vi "Process.vi"(0 "reference in":refnum<class "Reporter.lvclass">, 5 "error in (no error)":errorcluster) -> (14 "reference out":refnum<class "Reporter.lvclass">, 19 "error out":errorcluster)   [LabVIEW 2018, in "Reporter.lvclass"]
uses:
  Reporter.lvclass
  controls/IO Signal List.ctl
  BKP-891 LCR Meter_class/BKP-891 LCR Meter.lvclass
  BKP-911x Power Supply_class/BKP-911x Power Supply.lvclass
  NI-DAQmx_class/NI-DAQmx.lvclass
panel:
  in  "Signal MCLB":i32(listbox)
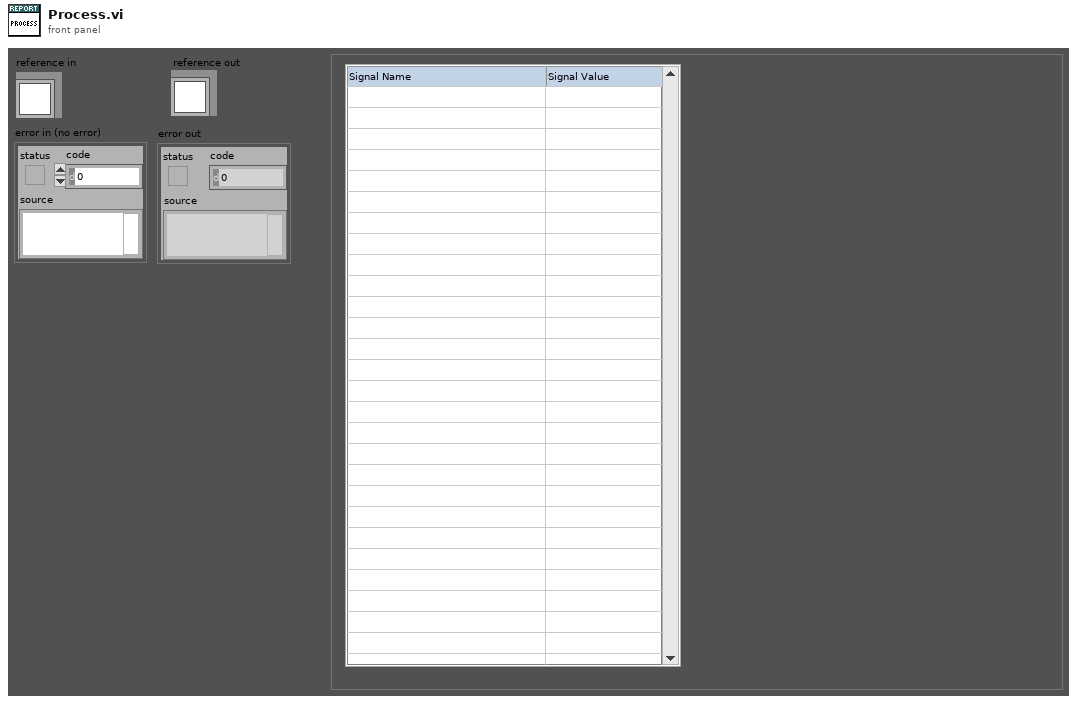
[diagram p1: front panel]
types:
  T1 = typedef "IO Signal List.ctl" = enum16{"Timestamp", "PSU_FB_U_VDC", "PSU_FB_I_AMP", "PSU_FB_W_WATT", "PSU_CMD_U_VDC", "PSU_CMD_I_AMP", "PSU_CMD_OUTPUT", "LCR_PRIMARY", "LCR_SECONDARY", "UV_R_mOhm", "UW_R_mOhm", "VW_R_mOhm", "UV_L_µH", "UW_L_µH", "VW_L_µH", "U_U_VDC", "V_U_VDC", "W_U_VDC", "U_I_AMP", "V_I_AMP", "W_I_AMP", "PWM_CMD_DC_%", "PWM_CMD_VDC", "PWM_CMD_Hz", "PWM_FB_DC_%", "PWM_FB_VDC", "PWM_FB_Hz", "DO_RELAY_U_LCR_A", "DO_RELAY_V_LCR_A", "DO_RELAY_V_LCR_B", "DO_RELAY_W_LCR_B", "DIFF_UV_UW_L_µH", "DIFF_UV_VW_L_µH", "DIFF_UW_VW_L_µH", "DIFF_UV_UW_R_mOhm", "DIFF_UV_VW_R_mOhm", "DIFF_UW_VW_R_mOhm", "DIFF_UV_U_VDC", "DIFF_UW_U_VDC", "DIFF_VW_U_VDC"}
  T2 = cluster{"Event":refnum<event-registration>, "Command":string, "Data":variant}
  T3 = typedef "Reporter.lvclass/ObjectAttributes.ctl" = cluster{"LCR":refnum<class "BKP-891 LCR Meter.lvclass">, "PSU":refnum<class "BKP-911x Power Supply.lvclass">, "NI-DAQmx":refnum<class "NI-DAQmx.lvclass">, "Signal List":T1[], "Latest Values":dbl[], "All Latest Values":dbl[], "All Signal List":T1[], "Report Directory":path, "Report File Ref":refnum<file>}
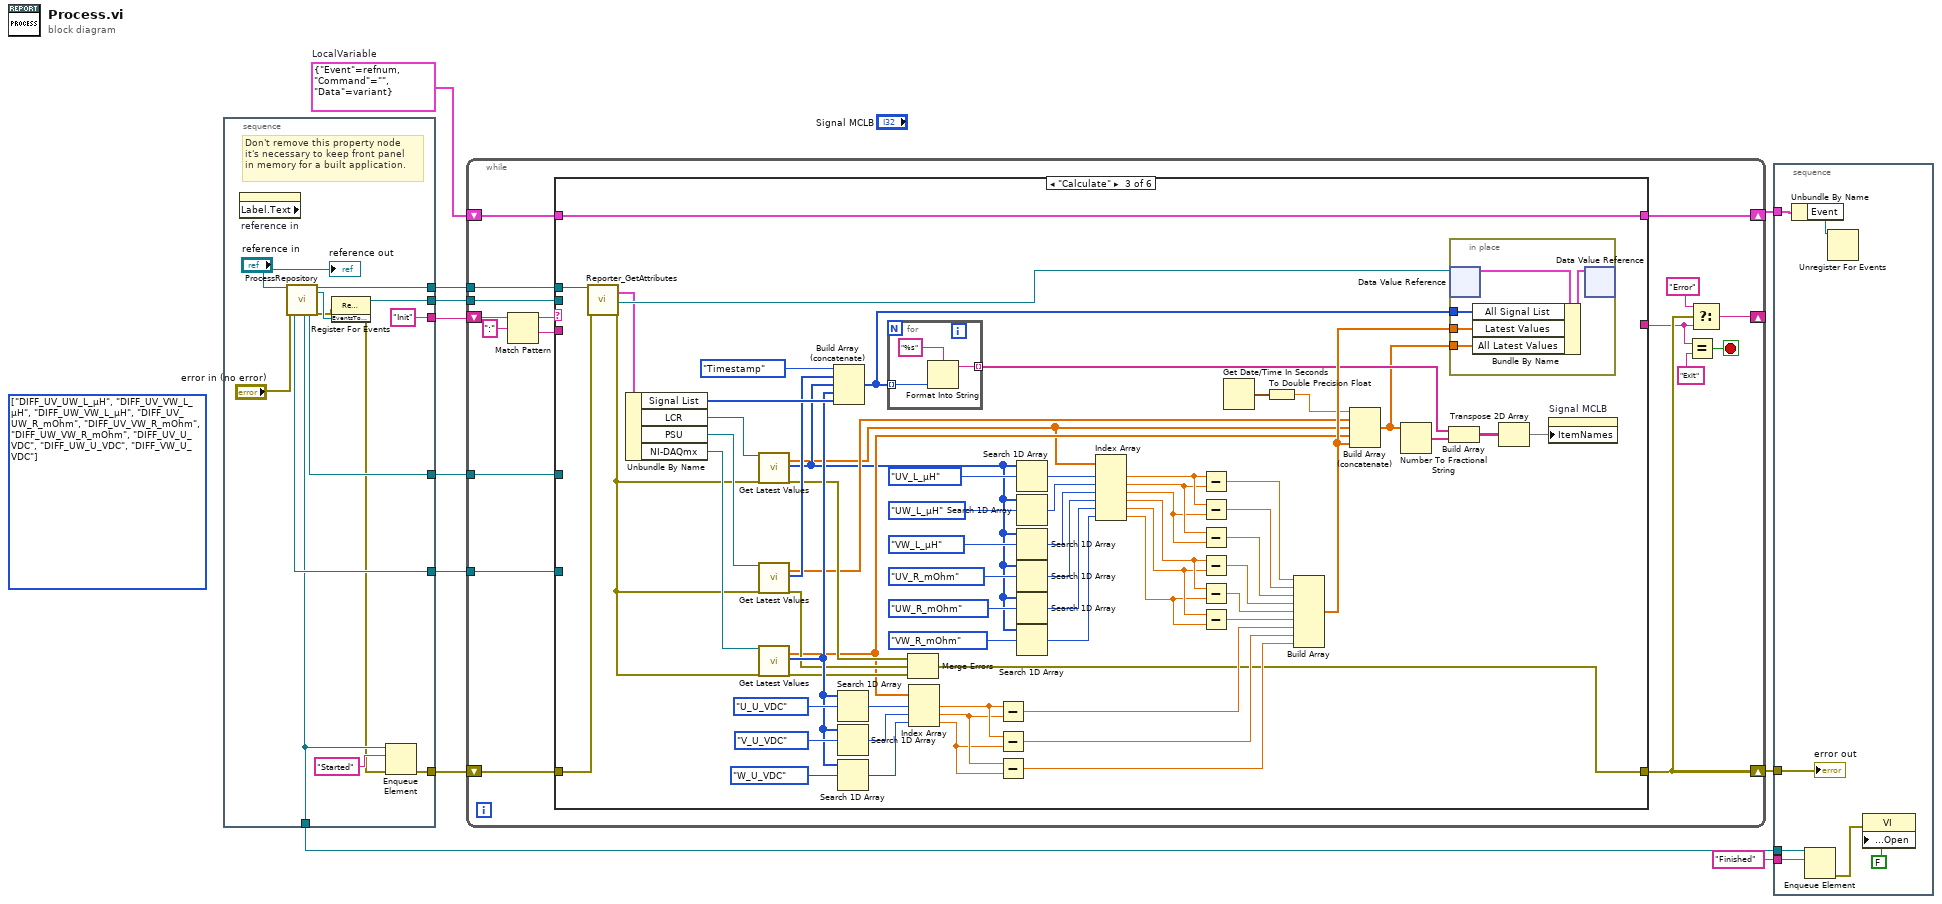
[diagram p0: block diagram]
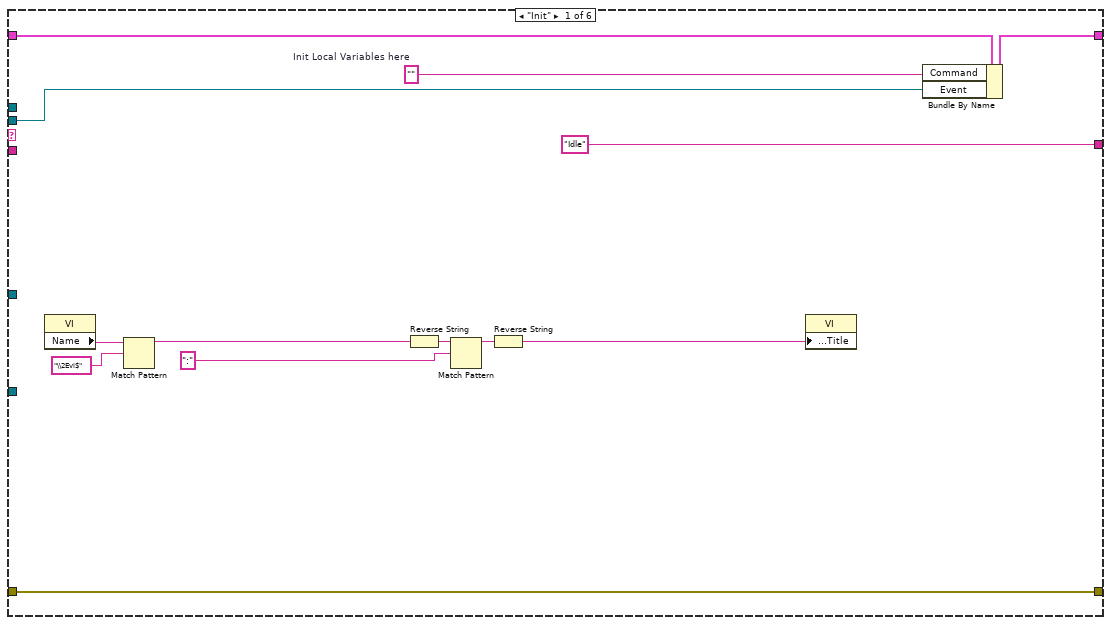
[diagram p2: hidden frame]
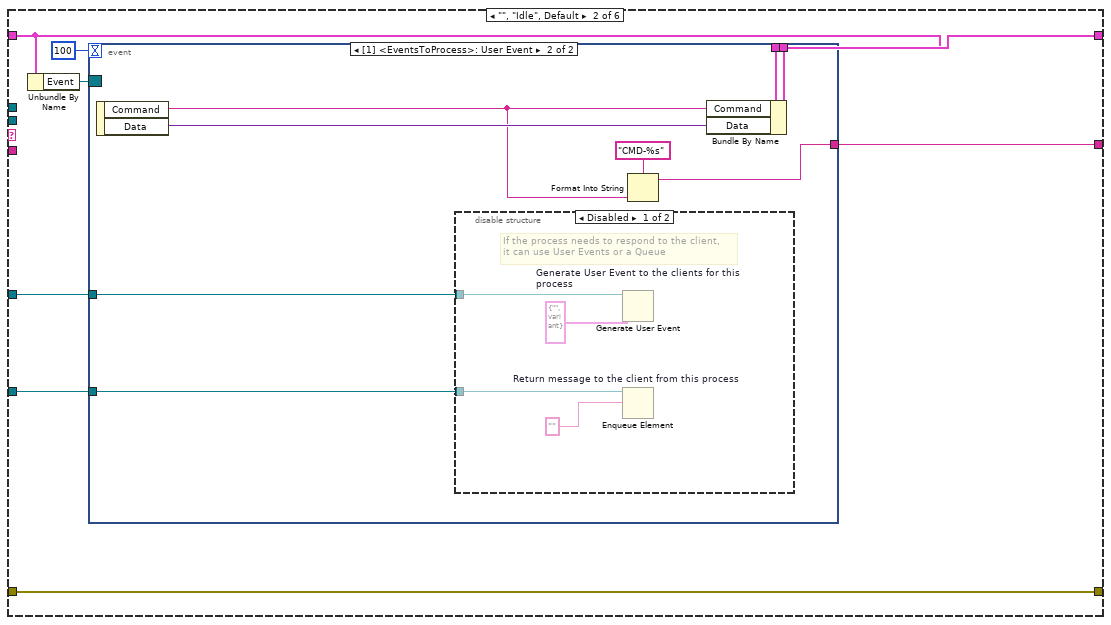
[diagram p3: hidden frame]
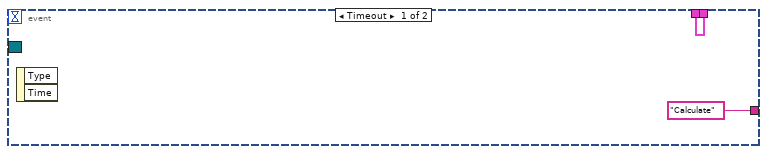
[diagram p4: hidden frame]
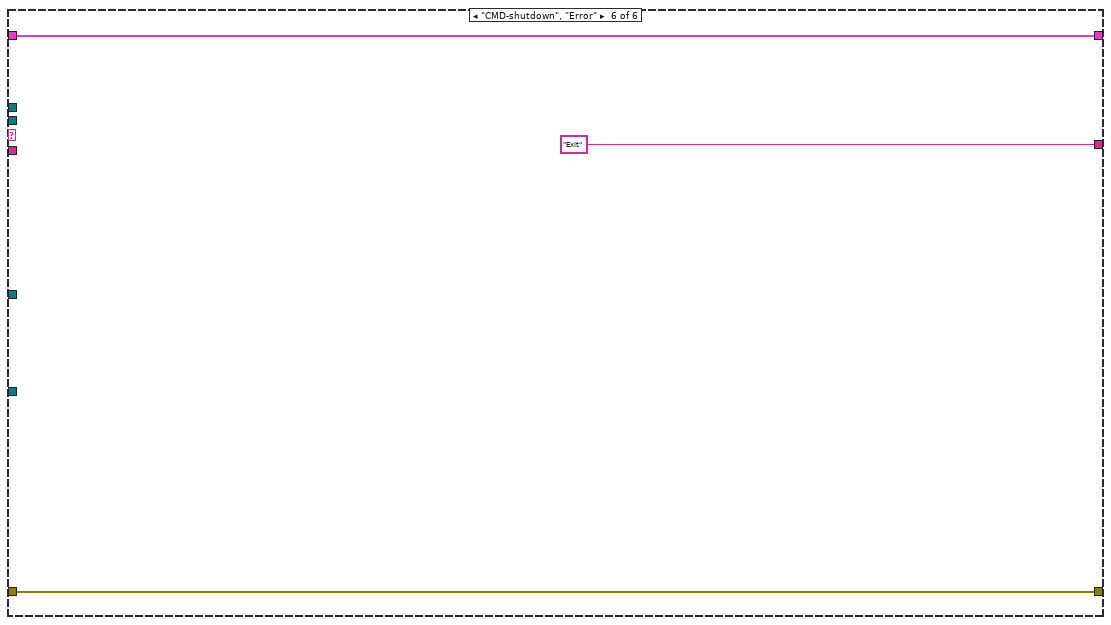
[diagram p8: hidden frame]
diagram:
  (unwired) T1[] [enum."DIFF_UV_UW_L_µH", enum."DIFF_UV_VW_L_µH", enum."DIFF_UW_VW_L_µH", enum."DIFF_UV_UW_R_mOhm", enum."DIFF_UV_VW_R_mOhm", enum."DIFF_UW_VW_R_mOhm", enum."DIFF_UV_U_VDC", enum."DIFF_UW_U_VDC", enum."DIFF_VW_U_VDC"] items=["Timestamp", "PSU_FB_U_VDC", "PSU_FB_I_AMP", "PSU_FB_W_WATT", "PSU_CMD_U_VDC", "PSU_CMD_I_AMP", "PSU_CMD_OUTPUT", "LCR_PRIMARY", "LCR_SECONDARY", "UV_R_mOhm", "UW_R_mOhm", "VW_R_mOhm", "UV_L_µH", "UW_L_µH", "VW_L_µH", "U_U_VDC", "V_U_VDC", "W_U_VDC", "U_I_AMP", "V_I_AMP", "W_I_AMP", "PWM_CMD_DC_%", "PWM_CMD_VDC", "PWM_CMD_Hz", "PWM_FB_DC_%", "PWM_FB_VDC", "PWM_FB_Hz", "DO_RELAY_U_LCR_A", "DO_RELAY_V_LCR_A", "DO_RELAY_V_LCR_B", "DO_RELAY_W_LCR_B", "DIFF_UV_UW_L_µH", "DIFF_UV_VW_L_µH", "DIFF_UW_VW_L_µH", "DIFF_UV_UW_R_mOhm", "DIFF_UV_VW_R_mOhm", "DIFF_UW_VW_R_mOhm", "DIFF_UV_U_VDC", "DIFF_UW_U_VDC", "DIFF_VW_U_VDC"]
  w1 = T2 {"Event"=refnum, "Command"="", "Data"=variant}  # LocalVariable
  n1 = stacked-sequence {
    tunnel: [w17] -> w11
    tunnel: [w24] -> w9
    tunnel: [w14] -> w8
    tunnel: [w18] -> w7
    tunnel: ["Init"] -> w6
    tunnel: [w20] -> w4
    tunnel: [w19] -> w3
    frame #0 {
      # "Don't remove this property node\nit's necessary to keep front panel\nin memory for a built application."
      n2 = property on="reference in" class="LVClassControl (strict)" props=["Label", "Text"]() -> ()  [unwired: 2 in, 3 out]
      n3 = call "ProcessRepository.vi"("reference in"="reference in", "error in (no error)"="error in (no error)") -> ("QueueFromProcess"=w19:refnum<queue>, "ProcessSyncQueue"=w18:refnum<queue>, "EventFromProcess"=w20:refnum<user-event>, "reference out"=w24:refnum<class "Reporter.lvclass">, "EventsToProcess"=w15:refnum<user-event>, "error out"=w13:errorcluster)  [unwired: 10 in, 2 out]
      n4 = register-events(error in=w13, w15) -> (reference out=w14:refnum<event-registration>, error out=w12:errorcluster)  [unwired: 1 in]
      n5 = Enqueue Element(queue=w18, element="Started", error in (no error)=w12) -> (error out=w17:errorcluster)  [unwired: 1 in, 2 out]
      "reference out" <- "reference in"
    }
  }
  n6 = while {
    shift-right: [w34] -> w10
    shift-left: w11 -> [w39]
    tunnel: w9 -> [w40]
    tunnel: w8 -> [w41]
    shift-right: [w32] -> _
    shift-left: w6 -> [w37]
    shift-right: [w28] -> w5
    shift-left: w1 -> [w27]
    tunnel: w4 -> [w26]
    tunnel: w3 -> [w25]
    stop <- w29 stop-if-true
    n7 = Match Pattern(string=w37, regular expression=":") -> (before substring=w36:string, after substring=w35:string)  [unwired: 1 in, 2 out]
    n8 = case shown="\"Calculate\"" w36 {
      tunnel: w39 -> [w52 w57 w140 w152 w154 w157]
      tunnel: [w52 w57 w112 w152 w154 w157] -> w34
      tunnel: w41 -> [w43 _ _ _ _ _]
      tunnel: w40 -> [_ _ w141 _ _ _]
      tunnel: w35 -> [_ _ _ _ _ _]
      tunnel: ["Idle" ("t") w62 _ _ _ "Exit" ("y")] -> w31
      tunnel: [w54 w61 w142 w151 w153 w155] -> w28
      tunnel: w27 -> [w42 w60 w142 w151 w153 w155]
      tunnel: w26 -> [_ w56 _ _ _ _]
      tunnel: w25 -> [_ w55 _ _ _ _]
      frame "Init" {
        w53 = ""  # Init Local Variables here
        n9 = property class="VI"() -> ("Name"=w50:string)  [unwired: 2 in, 2 out]
        n10 = Match Pattern(string=w50, regular expression="\\2Evi$") -> (before substring=w48:string)  [unwired: 1 in, 3 out]
        n11 = Reverse String(1:w48) -> (0:w47:string)
        n12 = Match Pattern(string=w47, regular expression=":") -> (before substring=w45:string)  [unwired: 1 in, 3 out]
        n13 = Reverse String(1:w45) -> (0:w44:string)
        n14 = property class="VI"("Front Panel.Title"=w44) -> ()  [unwired: 2 in, 2 out]
        n15 = Bundle By Name(cluster=w42, "Command"=w53, "Event"=w43) -> (w54:T2)
      }
      frame "", "Idle", Default {
        n16 = Unbundle By Name(w60) -> ("Event"=w59:refnum<event-registration>)
        n17 = event shown="[1] <EventsToProcess>: User Event" {
          selector: w59 -> [_ _]
          dyn-events: _ -> [_ _]
          timeout: 100 -> [_ _]
          tunnel: ["Calculate" ("t") w65] -> w62
          tunnel: w60 -> [w63 w72]
          tunnel: [w63 w71] -> w61
          tunnel: w56 -> [_ w67]
          tunnel: w55 -> [_ w66]
          event Timeout {
            n18 = event-data() -> ()  [unwired: 1 in, 2 out]
          }
          event User Event {
            n19 = event-data() -> ("Command"=w68:string, "Data"=w70:variant)  [unwired: 1 in]
            n20 = disable-structure shown="Disabled" {
              disable-tunnel: w67 -> [w76 _]
              disable-tunnel: w66 -> [w75 _]
              frame Disabled {
                # "If the process needs to respond to the client,\nit can use User Events or a Queue"
                n21 = Generate User Event "Generate User Event to the clients for this process"(user event=w76, event data cluster=cluster{"Command":string, "Data":variant} {"Command"="", "Data"=variant} ("event data")) -> ()  [unwired: 2 in, 2 out]
                n22 = Enqueue Element "Return message to the client from this process"(queue=w75, element="") -> ()  [unwired: 2 in, 3 out]
              }
              frame Enabled {
              }
            }
            n23 = Format Into String(format string="CMD-%s", w68) -> (resulting string=w65:string)  [unwired: 2 in, 1 out]
            n24 = Bundle By Name(cluster=w72, "Command"=w68, "Data"=w70) -> (w71:T2)
          }
        }
      }
      frame "Calculate" {
        n25 = call "Reporter_GetAttributes.vi"("reference in"=w141, "error in (no error)"=w140) -> ("Data"=w138:T3, "DataRef"=w139:refnum<data-value>, "error out"=w121:errorcluster)  [unwired: 14 in, 1 out]
        n26 = Unbundle By Name(w138) -> ("Signal List"=w125:T1[], "LCR"=w120:refnum<class "BKP-891 LCR Meter.lvclass">, "PSU"=w124:refnum<class "BKP-911x Power Supply.lvclass">, "NI-DAQmx"=w123:refnum<class "NI-DAQmx.lvclass">)
        n27 = call-dynamic "Get Latest Values.vi"("reference in"=w120, "error in (no error)"=w121) -> ("Latest Values"=w100:dbl[], "Signal List"=w101:T1[], "error out"=w116:errorcluster)  [unwired: 14 in, 1 out]
        n28 = call-dynamic "Get Latest Values.vi"("reference in"=w124, "error in (no error)"=w121) -> ("Latest Values"=w114:dbl[], "Signal List"=w119:T1[], "error out"=w115:errorcluster)  [unwired: 14 in, 1 out]
        n29 = call-dynamic "Get Latest Values.vi"("reference in"=w123, "error in (no error)"=w121) -> ("Latest Values"=w113:dbl[], "Signal List"=w122:T1[], "error out"=w117:errorcluster)  [unwired: 14 in, 1 out]
        n30 = Build Array (concatenate)(IO_Signal_List."Timestamp" ("IO Signal List"), w119, w101, w122, w125) -> (w78:T1[])
        n31 = Search 1D Array(1D array=w122, element=IO_Signal_List."U_U_VDC" ("IO Signal List")) -> (index of element=w134:i32)  [unwired: 1 in]
        n32 = Search 1D Array(1D array=w122, element=IO_Signal_List."V_U_VDC" ("IO Signal List")) -> (index of element=w133:i32)  [unwired: 1 in]
        n33 = Search 1D Array(1D array=w122, element=IO_Signal_List."W_U_VDC" ("IO Signal List")) -> (index of element=w132:i32)  [unwired: 1 in]
        n34 = for {
          tunnel: w78 -> [w145] mode=indexing
          tunnel: [w143] -> w105 mode=indexing
          n35 = Format Into String(format string="%s", w145) -> (resulting string=w143:string)  [unwired: 2 in, 1 out]
        }
        n36 = Merge Errors(w116, w115, w117) -> (w112:errorcluster)
        n37 = Index Array(array=w113, index #1=w134, index #2=w133, index #3=w132) -> (element #1=w131:dbl, element #2=w130:dbl, element #3=w129:dbl)
        n38 = Subtract(x=w131, y=w130) -> (x-y=w126:dbl)
        n39 = Subtract(x=w131, y=w129) -> (x-y=w127:dbl)
        n40 = Subtract(x=w130, y=w129) -> (x-y=w128:dbl)
        n41 = Search 1D Array(1D array=w101, element=IO_Signal_List."UV_L_µH" ("IO Signal List")) -> (index of element=w99:i32)  [unwired: 1 in]
        n42 = Search 1D Array(1D array=w101, element=IO_Signal_List."UW_L_µH" ("IO Signal List")) -> (index of element=w98:i32)  [unwired: 1 in]
        n43 = Search 1D Array(1D array=w101, element=IO_Signal_List."UV_R_mOhm" ("IO Signal List")) -> (index of element=w96:i32)  [unwired: 1 in]
        n44 = Search 1D Array(1D array=w101, element=IO_Signal_List."VW_L_µH" ("IO Signal List"), start index (0)=w96) -> (index of element=w97:i32)
        n45 = Search 1D Array(1D array=w101, element=IO_Signal_List."UW_R_mOhm" ("IO Signal List")) -> (index of element=w95:i32)  [unwired: 1 in]
        n46 = Search 1D Array(1D array=w101, element=IO_Signal_List."VW_R_mOhm" ("IO Signal List")) -> (index of element=w94:i32)  [unwired: 1 in]
        n47 = Index Array(array=w100, index #1=w99, index #2=w98, index #3=w97, index #4=w96, index #5=w95, index #6=w94) -> (element #1=w93:dbl, element #2=w92:dbl, element #3=w91:dbl, element #4=w90:dbl, element #5=w89:dbl, element #6=w88:dbl)
        n48 = Subtract(x=w93, y=w92) -> (x-y=w82:dbl)
        n49 = Subtract(x=w93, y=w91) -> (x-y=w83:dbl)
        n50 = Subtract(x=w92, y=w91) -> (x-y=w84:dbl)
        n51 = Subtract(x=w90, y=w89) -> (x-y=w85:dbl)
        n52 = Subtract(x=w90, y=w88) -> (x-y=w86:dbl)
        n53 = Subtract(x=w89, y=w88) -> (x-y=w87:dbl)
        n54 = Get Date/Time In Seconds() -> (seconds since 1Jan1904=w80:timestamp)
        n55 = To Double Precision Float(number=w80) -> (double precision float=w79:dbl)
        n56 = Build Array(w82, w83, w84, w85, w86, w87, w126, w127, w128) -> (w118:dbl[])
        n57 = Build Array (concatenate)(w79, w114, w100, w113, w118) -> (w81:dbl[])
        n58 = Number To Fractional String(number=w81) -> (F-format string=w111:string[])  [unwired: 3 in]
        n59 = Build Array(w105, w111) -> (w107:string[][])
        n60 = in-place {
          in-place-border: w118 -> [w148]
          in-place-border: w81 -> [w147]
          in-place-border: w78 -> [w146]
          n61 = in-place-dvr #1(w139) -> (w150:T3)  [unwired: 1 out]
          n62 = Bundle By Name(cluster=w150, "All Signal List"=w146, "Latest Values"=w148, "All Latest Values"=w147) -> (w149:T3)
          n63 = in-place-dvr #1(w149) -> ()  [unwired: 2 out]
        }
        n64 = Transpose 2D Array(2D array=w107) -> (transposed array=w106:string[][])
        n65 = property on="Signal MCLB" class="MCListbox (strict)"("ItemNames"=w106) -> ()  [unwired: 2 in, 2 out]
      }
      frame "---- COMMANDS START----" {
      }
      frame "----- COMMANDS END ----" {
      }
      frame "CMD-shutdown", "Error" {
      }
    }
    n66 = Equal?(x=w31, y="Exit") -> (x = y?=w29:bool)
    n67 = Select(t="Error", s=w34, f=w31) -> (s? t:f=w32:string)
  }
  n68 = stacked-sequence {
    tunnel: w10 -> [w164]
    tunnel: w7 -> [w160]
    tunnel: w5 -> [w163]
    tunnel: "Finished" ("element") -> [w158]
    frame #0 {
      n69 = Unbundle By Name(w163) -> ("Event"=w162:refnum<event-registration>)
      n70 = Enqueue Element(queue=w160, element=w158) -> (error out=w159:errorcluster)  [unwired: 2 in, 2 out]
      n71 = Unregister For Events(event registration refnum=w162) -> ()  [unwired: 1 in, 1 out]
      n72 = property class="VI"(error in=w159, "Front Panel.Open"=FALSE ("Front Panel Window:Open")) -> ()  [unwired: 1 in, 2 out]
      "error out" <- w164
    }
  }
